vi "数据转JOSN发送.vi"() -> ()   [LabVIEW 2016, in "工况数据上传.lvlib"]
uses:
  <vilib>/httpClient/POSTBuffer.vi
  <vilib>/httpClient/LabVIEWHTTPClient.lvlib
panel:
  out "元素":string
  out "body":string caption="体部"
  out "headers":string caption="头部"
  out "error out":errorcluster
  out "time":string="2021-05-08 14:02:02"
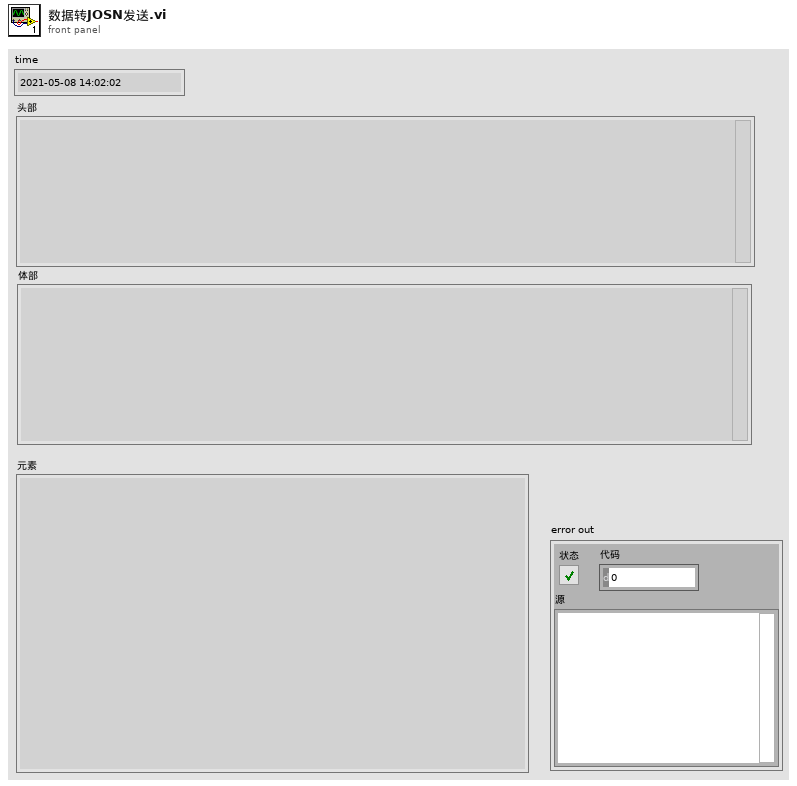
[diagram p1: front panel]
types:
  T1 = cluster{"url":string, "loginTokenRequest":cluster{"clientId":string, "clientSecret":string, "grantType":string, "password":string, "scope":string, "userName":string, "userType":string}, "自动获取MN":bool}
  T2 = typedef "工况数据.ctl" = cluster{"time":string, "data":cluster{"ups":cluster{"ups":cluster{"input_voltage":ext, "input_frequency":ext, "output_voltage":ext, "output_current":ext, "output_frequency":ext, "output_active_power":ext, "output_apparent_power":ext, "load_rate":ext, "cabinet_temperature":ext, "battery_voltage":ext, "remaining_battery_capacity":ext, "power_on_status":string, "power_supply_mode":string, "fault":bool, "battery_low_voltage":bool, "mains_supply_abnormality":bool}, "启用":bool}, "air_conditioner":cluster{"air_conditioner":cluster{"cabinet_temperature":ext, "air_supply_temperature":ext, "voltage":ext, "current":ext, "compressor_status":string, "Internal_fan_status":string, "external_fan_status":string, "heating_state":string, "refrigeration_state":bool, "high_temperature_alarm":bool, "low_temperature_alarm":bool, "heater_fault":bool, "temperature_sensor_fault":bool, "high_voltage_alarm":bool, "low_voltage_alarm":bool, "refrigeration_start_point":ext, "refrigeration_sensitive_point":ext, "heating_start_point":ext, "heating_sensitive_point":ext, "high_temperature_alarm_point":ext, "low_temperature_alarm_point":ext}, "启用":bool}, "smoke_sensor":cluster{"smoke_sensor":cluster{"trigger_alarm":bool}, "启用":bool}, "water_immersion_sensor":cluster{"water_immersion_sensor":cluster{"trigger_alarm":bool}, "启用":bool}, "temperature_and_humidity_sensor":cluster{"temperature_and_humidity_sensor":cluster{"current_temperature":ext, "current_humidity":ext, "room_temperature_alarm":bool, "humidity_alarm":bool}, "启用":bool}, "gps":cluster{"gps":cluster{"current_longitude":ext, "current_latitude":ext, "launch_longitude":ext, "launch_latitude":ext, "shift_alarm":bool}, "启用":bool}, "solar_controller":cluster{"solar_controller":cluster{"array_voltage":ext, "array_current":ext, "generating_power":ext, "battery_voltage":dbl, "battery_current":ext, "ceiling_voltage":ext, "minimum_voltage":ext, "battery_temperature":ext, "remaining_battery_capacity":ext, "load_voltage":ext, "load_current":ext, "load_power":ext, "equipment_temperature":ext, "accumulated_electricity_consumption_of_the_day":ext, "accumulated_electricity_consumption_of_the_current_month":ext, "accumulated_electricity_consumption_in_the_current_year":ext, "total_accumulated_power_consumption":ext, "accumulated_charging_capacity_of_the_day":ext, "accumulated_charging_amount_of_the_current_month":ext, "accumulated_charging_capacity_of_the_current_year":ext, "total_cumulative_charge":ext}, "启用":bool}, "solar_controller_2":cluster{"solar_controller_2":cluster{"array_voltage":ext, "array_current":ext, "generating_power":ext, "battery_voltage":dbl, "battery_current":ext, "ceiling_voltage":ext, "minimum_voltage":ext, "battery_temperature":ext, "remaining_battery_capacity":ext, "load_voltage":ext, "load_current":ext, "load_power":ext, "equipment_temperature":ext, "accumulated_electricity_consumption_of_the_day":ext, "accumulated_electricity_consumption_of_the_current_month":ext, "accumulated_electricity_consumption_in_the_current_year":ext, "total_accumulated_power_consumption":ext, "accumulated_charging_capacity_of_the_day":ext, "accumulated_charging_amount_of_the_current_month":ext, "accumulated_charging_capacity_of_the_current_year":ext, "total_cumulative_charge":ext}, "启用":bool}}}
  T3 = cluster{"code":string, "message":string, "timestamp":u64, "data":cluster{"bearerType":string, "oauth2Type":string, "accessToken":string, "tokenType":string, "expiresIn":u64, "refreshToken":string, "scope":string[], "tokenDetail":cluster{"dataSource":string, "username":string, "userId":string, "userType":string, "enabled":bool, "accountNonExpired":bool, "credentialsNonExpired":bool, "accountNonLocked":bool}}, "success":bool}
  T4 = typedef "LabVIEWHTTPClient.lvlib/ClientHandle.ctl" = refnum<k1>
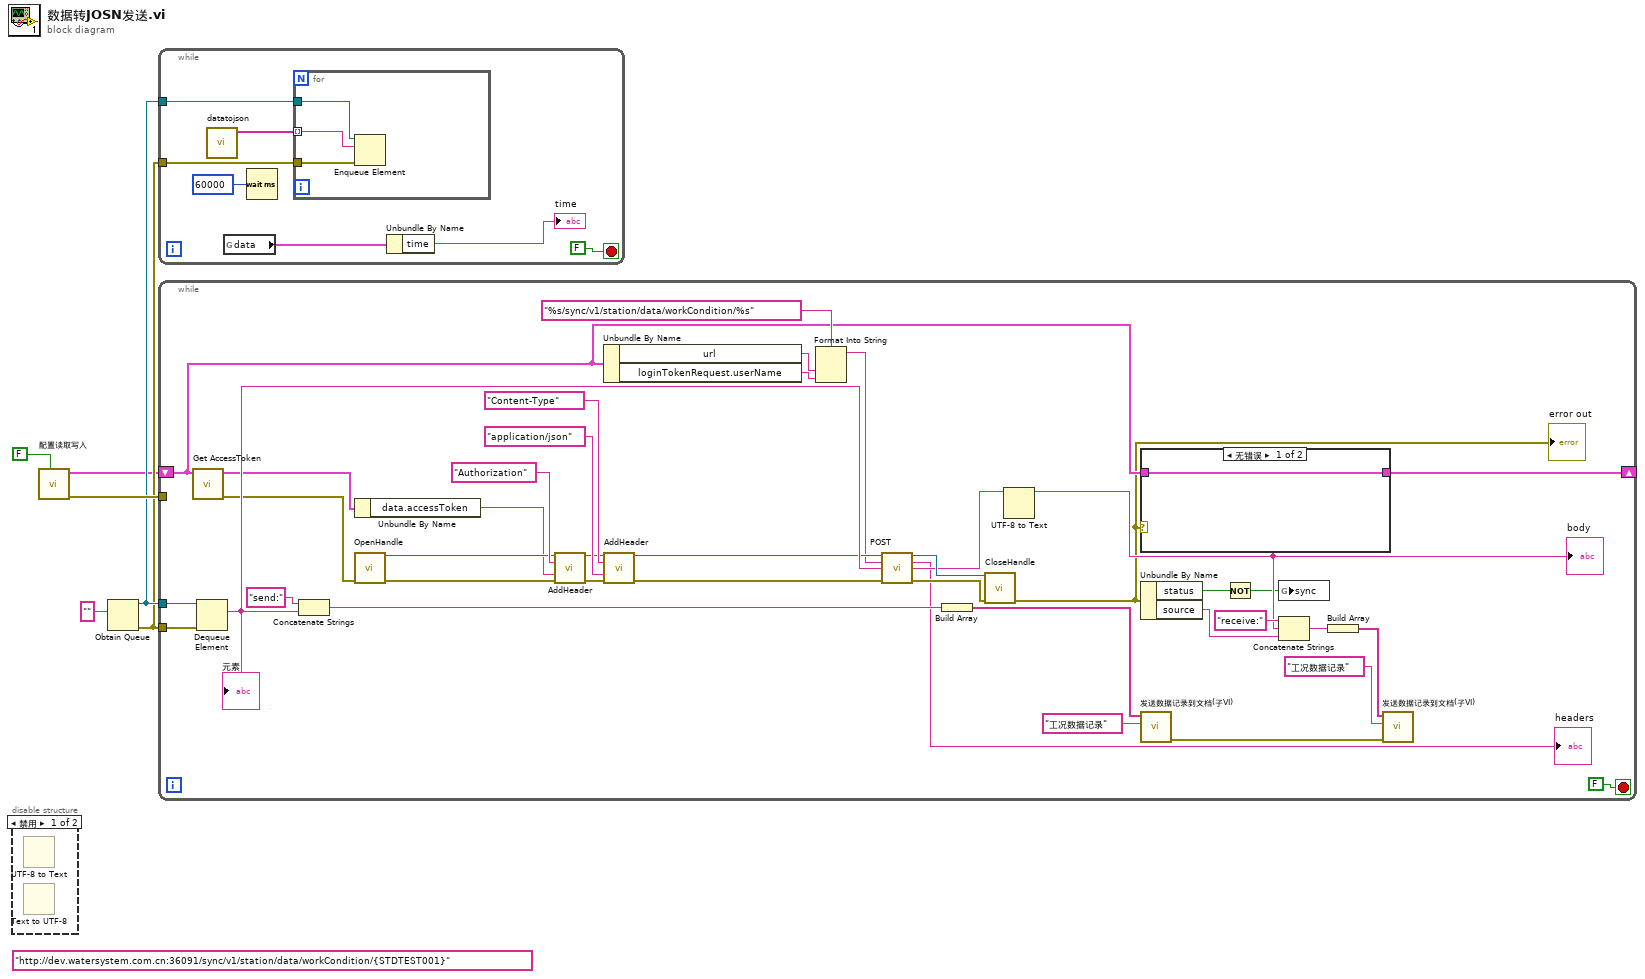
[diagram p0: block diagram]
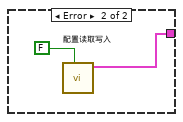
[diagram p2: hidden frame]
diagram:
  (unwired) "http://dev.watersystem.com.cn:36091/sync/v1/station/data/workCondition/{STDTEST001}"
  n1 = disable-structure shown="禁用" {
    frame Disabled {
      n2 = UTF-8 to Text() -> ()  [unwired: 3 in, 2 out]
      n3 = Text to UTF-8() -> ()  [unwired: 3 in, 2 out]
    }
    frame Enabled {
    }
  }
  n4 = call "配置读取写入.vi"("write"=FALSE) -> ("error out"=w4:errorcluster, "配置输出"=w1:T1)  [unwired: 9 in]
  n5 = Obtain Queue(element data type="") -> (queue out=w3:refnum<queue>, error out=w2:errorcluster)  [unwired: 4 in, 1 out]
  n6 = while {
    tunnel: w3 -> [w11]
    tunnel: w2 -> [w10]
    stop <- FALSE stop-if-true
    n7 = call "datatojson.vi"() -> ("json"=w7:string[])  [unwired: 11 in]
    n8 = global read "工况数据接口全局.vi" "data"() -> (w8:T2)
    n9 = Wait (ms)(milliseconds to wait=u32 60000 ("等待时间（毫秒）")) -> ()  [unwired: 1 out]
    n10 = for {
      tunnel: w11 -> [w16]
      tunnel: w10 -> [w15]
      tunnel: w7 -> [w14] mode=indexing
      n11 = Enqueue Element(queue=w16, element=w14, error in (no error)=w15) -> ()  [unwired: 1 in, 3 out]
    }
    n12 = Unbundle By Name(w8) -> ("time"=→"time":string)
  }
  n13 = while {
    tunnel: w3 -> [w50]
    tunnel: w2 -> [w49]
    tunnel: w4 -> [_]
    shift-right: [w22] -> _
    shift-left: w1 -> [w21]
    stop <- FALSE stop-if-true
    n14 = call "Get AccessToken.vi"("配置"=w21) -> ("error out"=w36:errorcluster, "response"=w35:T3)  [unwired: 9 in]
    n15 = Dequeue Element(queue=w50, error in (no error)=w49) -> (element=w53:string)  [unwired: 1 in, 3 out]
    "元素" <- w53
    n16 = Concatenate Strings("send:" ("字符串"), w53) -> (w54:string)
    n17 = Unbundle By Name(w35) -> ("data.accessToken"=w34:string)
    n18 = call <vilib>:"OpenHandle.vi"("error in (no error)"=w36) -> ("client handle out"=w39:T4, "error out"=w38:errorcluster)  [unwired: 13 in]
    n19 = call <vilib>:"AddHeader.vi"("client handle"=w39, "header"="Authorization", "value"=w34, "error in (no error)"=w38) -> ("client handle out"=w40:T4, "error out"=w37:errorcluster)  [unwired: 10 in]
    n20 = Unbundle By Name(w21) -> ("url"=w32:string, "loginTokenRequest.userName"=w31:string)
    n21 = call <vilib>:"AddHeader.vi"("client handle"=w40, "header"="Content-Type", "value"="application/json", "error in (no error)"=w37) -> ("client handle out"=w43:T4, "error out"=w42:errorcluster)  [unwired: 10 in]
    n22 = Format Into String(format string="%s/sync/v1/station/data/workCondition/%s" ("url"), w32, w31) -> (resulting string=w30:string)  [unwired: 2 in, 1 out]
    n23 = call-poly <vilib>:"POST.vi"("client handle"=w43, "url"=w30, "buffer"=w53, "error in (no error)"=w42) -> ("client handle out"=w46:T4, "headers"=→"headers":string, "body"=w44:string, "error out"=w45:errorcluster)  [unwired: 8 in]
    n24 = Build Array(w54) -> (w52:string[])
    n25 = call <vilib>:"CloseHandle.vi"("client handle"=w46, "error in (no error)"=w45) -> ("error out"=w20:errorcluster)  [unwired: 13 in]
    "error out" <- w20
    n26 = UTF-8 to Text(11:w44) -> (3:w24:string)  [unwired: 2 in, 1 out]
    "body" <- w24
    n27 = case shown="无错误" w20 {
      tunnel: [w57 w58] -> w22
      tunnel: w21 -> [w57 _]
      frame No Error {
      }
      frame Error {
        n28 = call "配置读取写入.vi"("write"=FALSE) -> ("配置输出"=w58:T1)  [unwired: 9 in, 1 out]
      }
    }
    n29 = Unbundle By Name(w20) -> ("status"=w19:bool, "source"=w17:string)
    n30 = call "发送数据记录到文档(子VI).vi"("字符串"="工况数据记录", "数组"=w52) -> ("错误输出"=w23:errorcluster)  [unwired: 8 in]
    n31 = Not(x=w19) -> (.not. x?=w18:bool)
    n32 = global write "工况数据接口全局.vi" "sync"(w18) -> ()
    n33 = Concatenate Strings("receive:" ("字符串"), w24, w17) -> (w28:string)
    n34 = Build Array(w28) -> (w26:string[])
    n35 = call "发送数据记录到文档(子VI).vi"("错误输入"=w23, "字符串"="工况数据记录", "数组"=w26) -> ()  [unwired: 7 in, 1 out]
  }
